vi "Save Animated GIF To Memory (Core).vi"(7 "Dither (None)":T2, 8 "error in (no error)":errorcluster, 9 "Delays":i32[](array[numeric]), 10 "Frames":T1[](array[typedef])) -> (0 "error out":errorcluster, 3 "Encoded Image":u8[](array[numeric]))   [LabVIEW 2020, in "G-Image.lvlib"]
doc: "Saves an image in GIF format to disk."
uses:
  G-Image.lvlib
  lib/g_image_32.dll
  <vilib>/picture/picture.llb/imagedata.ctl
  Controls/Dither Type.ctl
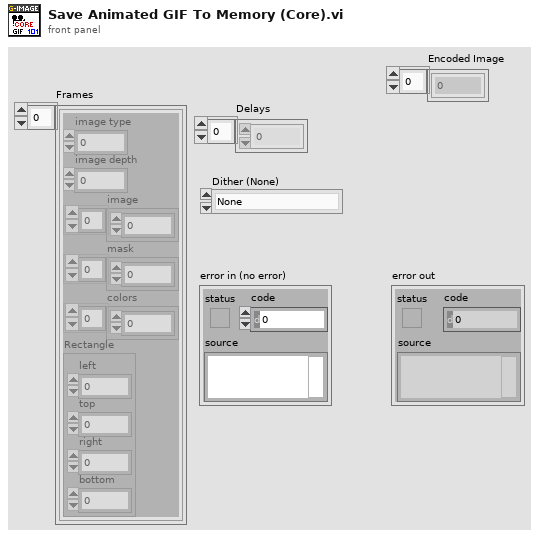
[diagram p1: front panel]
types:
  T1 = typedef "imagedata.ctl" = cluster{"image type":i32, "image depth":i32, "image":u8[], "mask":u8[], "colors":u32[], "Rectangle":cluster{"left":i16, "top":i16, "right":i16, "bottom":i16}}
  T2 = typedef "G-Image.lvlib/Dither Type.ctl" = enum32{"None", "Floyd-Steinberg"}
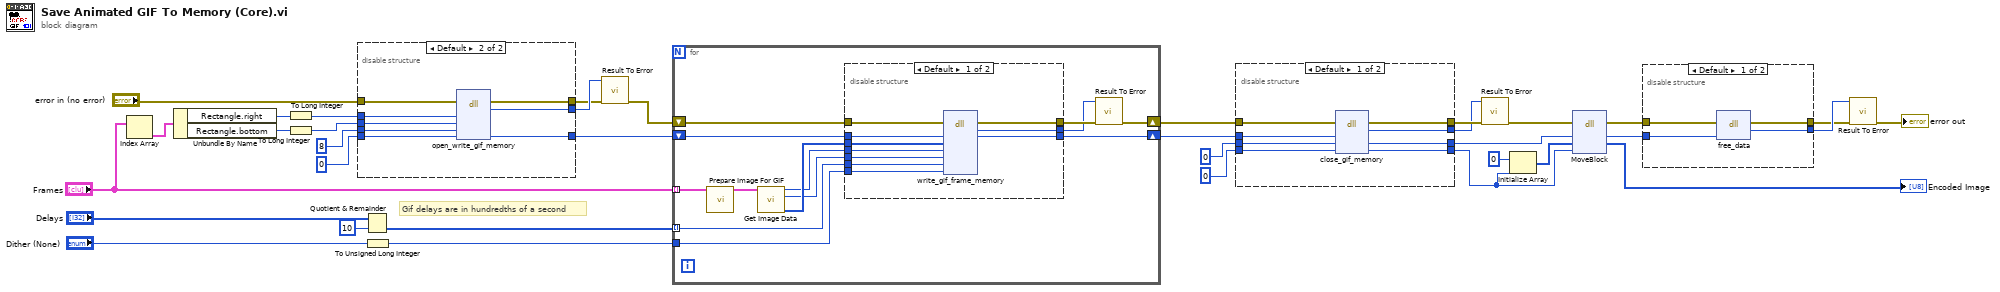
[diagram p0: block diagram]
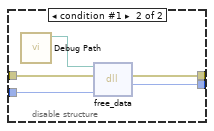
[diagram p2: hidden frame]
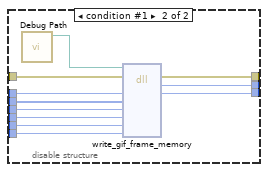
[diagram p3: hidden frame]
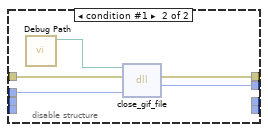
[diagram p4: hidden frame]
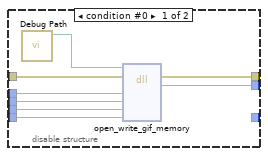
[diagram p5: hidden frame]
diagram:
  # "Gif delays are in hundredths of a second"
  n1 = Index Array(array="Frames") -> (element=w32:T1)  [unwired: 1 in]
  n2 = Unbundle By Name(w32) -> ("Rectangle.right"=w31:i16, "Rectangle.bottom"=w29:i16)
  n3 = To Long Integer(number=w31) -> (32bit integer=w30:i32)
  n4 = To Long Integer(number=w29) -> (32bit integer=w28:i32)
  n5 = disable-structure shown="Default" {
    disable-tunnel: [w43 w51] -> w33
    disable-tunnel: "error in (no error)" -> [w42 w50]
    disable-tunnel: [w41 w49] -> w34
    disable-tunnel: w30 -> [w39 w48]
    disable-tunnel: w28 -> [w38 w47]
    disable-tunnel: 8 -> [w37 w46]
    disable-tunnel: i64 0 ("writer_ptr") -> [w36 w45]
    disable-tunnel: [_ w44] -> w24
    frame condition #0 {
      n6 = call "Debug Path.vi"() -> ("Debug Path"=w40:path)  [unwired: 11 in]
      n7 = dll-call lib="?" fn="open_write_gif_memory"(path in=w40, error in=w42, "width"=w39, "height"=w38, "depth"=w37, "writer_ptr"=w36) -> (error out=w43:errorcluster, "result"=w41:i32)  [unwired: 5 in, 1 out]
    }
    frame condition #1 (active) {
      n8 = dll-call lib="C:/github/dataflowg/g-image/src/LabVIEW/G-Image/lib/g_image_*.*" fn="open_write_gif_memory"(error in=w50, "width"=w48, "height"=w47, "depth"=w46, "writer_ptr"=w45) -> (error out=w51:errorcluster, "result"=w49:i32, "writer_ptr"=w44:i64)  [unwired: 5 in, 1 out]
    }
  }
  n9 = Quotient & Remainder(x="Delays", y=10) -> (floor(x/y)=w14:i32[])  [unwired: 1 out]
  n10 = To Unsigned Long Integer(number="Dither (None)") -> (unsigned 32bit integer=w21:u32)
  n11 = call "Result To Error.vi"("error in (no error)"=w33, "Result Code"=w34) -> ("error out"=w20:errorcluster)  [unwired: 9 in]
  n12 = for {
    shift-right: [w63] -> w18
    shift-left: w24 -> [w64]
    tunnel: "Frames" -> [w56] mode=indexing
    tunnel: w14 -> [w62] mode=indexing
    tunnel: w21 -> [w61]
    shift-right: [w58] -> w19
    shift-left: w20 -> [w57]
    n13 = call "Prepare Image For GIF.vi"("Image"=w56) -> ("Image"=w55:T1)  [unwired: 9 in, 1 out]
    n14 = call "Get Image Data.vi"("Image"=w55) -> ("Image (RGBA)"=w54:u8[], "Height"=w52:i32, "Width"=w53:i32)  [unwired: 7 in, 1 out]
    n15 = disable-structure shown="Default" {
      disable-tunnel: [w74 w85] -> w60
      disable-tunnel: w57 -> [w73 w84]
      disable-tunnel: [w72 w83] -> w59
      disable-tunnel: w64 -> [w71 w82]
      disable-tunnel: w54 -> [w69 w80]
      disable-tunnel: w53 -> [w68 w79]
      disable-tunnel: w52 -> [w67 w78]
      disable-tunnel: w62 -> [w66 w77]
      disable-tunnel: [w70 w81] -> w63
      disable-tunnel: w61 -> [w65 w76]
      frame condition #0 (active) {
        n16 = dll-call lib="C:/github/dataflowg/g-image/src/LabVIEW/G-Image/lib/g_image_*.*" fn="write_gif_frame_memory"(error in=w73, "writer_ptr"=w71, "image_data"=w69, "width"=w68, "height"=w67, "delay"=w66, "dither"=w65) -> (error out=w74:errorcluster, "result"=w72:i32, "writer_ptr"=w70:i64)  [unwired: 7 in, 1 out]
      }
      frame condition #1 {
        n17 = call "Debug Path.vi"() -> ("Debug Path"=w75:path)  [unwired: 11 in]
        n18 = dll-call lib="?" fn="write_gif_frame_memory"(path in=w75, error in=w84, "writer_ptr"=w82, "image_data"=w80, "width"=w79, "height"=w78, "delay"=w77, "dither"=w76) -> (error out=w85:errorcluster, "result"=w83:i32, "writer_ptr"=w81:i64)  [unwired: 6 in, 1 out]
      }
    }
    n19 = call "Result To Error.vi"("error in (no error)"=w60, "Result Code"=w59) -> ("error out"=w58:errorcluster)  [unwired: 9 in]
  }
  n20 = disable-structure shown="Default" {
    disable-tunnel: [w93 w98] -> w17
    disable-tunnel: w19 -> [w92 w97]
    disable-tunnel: [w91 w96] -> w16
    disable-tunnel: w18 -> [w90 w95]
    disable-tunnel: i64 0 -> [w89 _]
    disable-tunnel: 0 -> [w88 _]
    disable-tunnel: [w87 _] -> w6
    disable-tunnel: [w86 _] -> w5
    frame condition #0 (active) {
      n21 = dll-call lib="C:/github/dataflowg/g-image/src/LabVIEW/G-Image/lib/g_image_*.*" fn="close_gif_memory"(error in=w92, "writer_ptr"=w90, "encoded_image"=w89, "encoded_image_count"=w88) -> (error out=w93:errorcluster, "result"=w91:i32, "encoded_image"=w87:i64, "encoded_image_count"=w86:i32)  [unwired: 3 in, 1 out]
    }
    frame condition #1 {
      n22 = call "Debug Path.vi"() -> ("Debug Path"=w94:path)  [unwired: 11 in]
      n23 = dll-call lib="?" fn="close_gif_file"(path in=w94, error in=w97, "writer_ptr"=w95) -> (error out=w98:errorcluster, "result"=w96:i32)  [unwired: 2 in, 1 out]
    }
  }
  n24 = call "Result To Error.vi"("error in (no error)"=w17, "Result Code"=w16) -> ("error out"=w4:errorcluster)  [unwired: 9 in]
  n25 = Initialize Array(u8 0 ("element"), w5) -> (w12:u8[])
  n26 = dll-call lib="LabVIEW" fn="MoveBlock"(error in=w4, "Address (Pointer)"=w6, "Destination"=w12, "Size"=w5) -> (error out=w3:errorcluster, "Address (Pointer)"=w10:i64, "Destination"=→"Encoded Image":u8[])  [unwired: 4 in, 1 out]
  n27 = disable-structure shown="Default" {
    disable-tunnel: w10 -> [w102 w107]
    disable-tunnel: w3 -> [w101 w106]
    disable-tunnel: [w100 w105] -> w9
    disable-tunnel: [w99 w104] -> w2
    frame condition #0 (active) {
      n28 = dll-call lib="C:/github/dataflowg/g-image/src/LabVIEW/G-Image/lib/g_image_*.*" fn="free_data"(error in=w101, "encoded_image"=w102) -> (error out=w99:errorcluster, "result"=w100:i32)  [unwired: 3 in, 1 out]
    }
    frame condition #1 {
      n29 = call "Debug Path.vi"() -> ("Debug Path"=w103:path)  [unwired: 11 in]
      n30 = dll-call lib="?" fn="free_data"(path in=w103, error in=w106, "encoded_image"=w107) -> (error out=w104:errorcluster, "result"=w105:i32)  [unwired: 2 in, 1 out]
    }
  }
  n31 = call "Result To Error.vi"("error in (no error)"=w2, "Result Code"=w9) -> ("error out"=→"error out":errorcluster)  [unwired: 9 in]
